vi "Wait for Idle.vi"(0 "VISA resource name":refnum<visa-resource-name>, 11 "error in (no error)":errorcluster) -> (4 "VISA resource name out":refnum<visa-resource-name>, 15 "error out":errorcluster)   [LabVIEW 2024, in "Keithley 648X Series.lvlib"]
doc: "Waits for the instrument to return to the idle state or experience an error."
uses:
  <instrlib>/Keithley 648X Series/Keithley 648X Series.lvlib
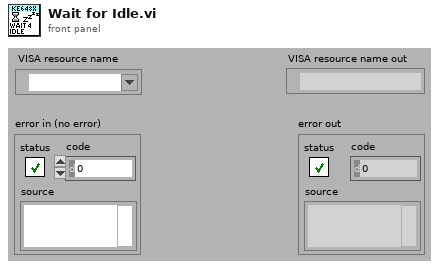
[diagram p1: front panel]
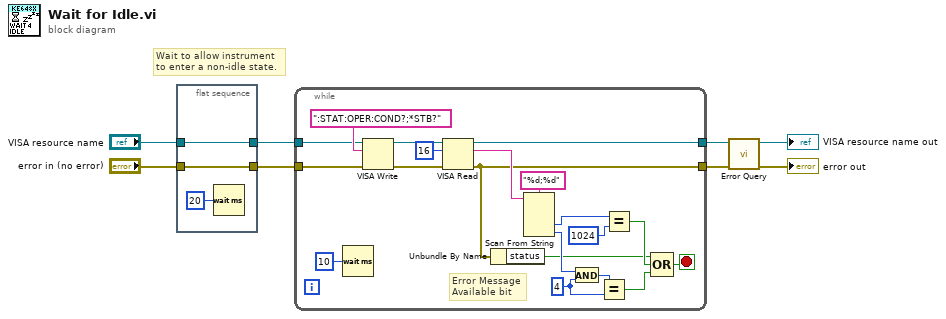
[diagram p0: block diagram]
diagram:
  # "Wait to allow instrument\nto enter a non-idle state."
  n1 = flat-sequence {
    tunnel: [w10] -> w7
    tunnel: "VISA resource name" -> [w10]
    tunnel: "error in (no error)" -> [w9]
    tunnel: [w9] -> w6
    frame #0 {
      n2 = Wait (ms)(milliseconds to wait=u32 20) -> ()  [unwired: 1 out]
    }
  }
  n3 = while {
    tunnel: w7 -> [w30]
    tunnel: w6 -> [w29]
    tunnel: [w15] -> w3
    tunnel: [w23] -> w4
    stop <- w13 stop-if-true
    w17 = 4 ("y")
    # "Error Message\nAvailable bit"
    n4 = Wait (ms)(milliseconds to wait=u32 10) -> ()  [unwired: 1 out]
    n5 = VISA Write(VISA resource name=w30, write buffer=":STAT:OPER:COND?;*STB?" ("Reset Command"), error in (no error)=w29) -> (VISA resource name out=w28:refnum<visa-resource-name>, error out=w27:errorcluster)  [unwired: 1 out]
    n6 = VISA Read(VISA resource name=w28, byte count=u32 16, error in (no error)=w27) -> (VISA resource name out=w23:refnum<visa-resource-name>, read buffer=w22:string, error out=w15:errorcluster)  [unwired: 1 out]
    n7 = Unbundle By Name(w15) -> ("status"=w12:bool)
    n8 = Scan From String(format string="%d;%d", input string=w22) -> (output 1=w20:i32, output 2=w19:i32)  [unwired: 4 in, 3 out]
    n9 = And(x=w19, y=w17) -> (x .and. y?=w18:i32)
    n10 = Equal?(x=w18, y=w17) -> (x = y?=w16:bool)
    n11 = Equal?(x=w20, y=1024) -> (x = y?=w14:bool)
    n12 = Compound Arithmetic op=OR(w12, w14, w16) -> (w13:bool)
  }
  n13 = call <instrlib>:"Error Query.vi"("error in (no error)"=w3, "VISA resource name"=w4) -> ("error out"=→"error out":errorcluster, "VISA resource name out"=→"VISA resource name out":refnum<visa-resource-name>)  [unwired: 6 in, 2 out]
